vi "Convert Array to ImprocOptions.vi"(1 "Array":i32[](array[numeric])) -> (0 "IMPROCOPTIONS":T1 {"FilterCode" items=["PREWITT_3X3_V"=1, "PREWITT_3X3_H"=2, "SOBEL_3X3_V"=3, "SOBEL_3X3_H"=4, "LAPLACIAN_3X3"=5, "LAPLACIAN_5X5"=6, "GAUSSIAN_3X3"=7, "GAUSSIAN_5X5"=8, "HIPASS_3x3"=9, "HIPASS_5x5"=10, "SHARPEN_3X3"=11, "USERFILTER"=-1]; "Rotate" min=-90 max=90 step=1; "Saturation" min=-100 max=100 step=1; "Contrast" min=-100 max=100 step=1; "Bright" min=-100 max=100 step=1})   [LabVIEW 2013, in "VRI.lvlib"]
uses:
  VRI.lvlib
  _Type Defs/PhInt IMPROCOPTIONS.ctl
  _Type Defs/PhInt WBGAIN.ctl
  _Type Defs/FilterCode.ctl
  _Type Defs/IMFILTER.ctl
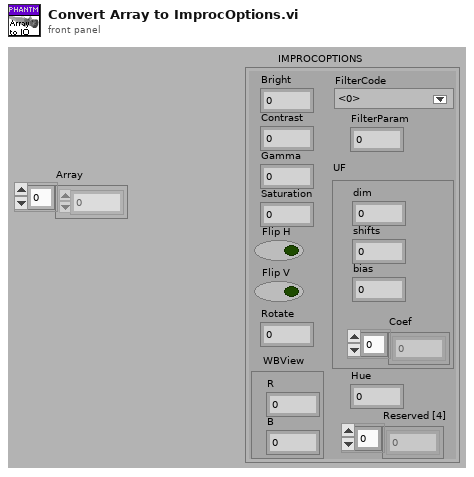
[diagram p1: front panel]
types:
  T1 = typedef "VRI.lvlib/PhInt IMPROCOPTIONS.ctl" = cluster{"Bright":i32, "Contrast":i32, "Gamma":sgl, "Saturation":i32, "Flip H":bool, "Flip V":bool, "Rotate":i32, "WBView":T2, "FilterCode":T3, "FilterParam":i32, "UF":T4, "Hue":i32, "Reserved [4]":i32[]}
  T2 = typedef "VRI.lvlib/PhInt WBGAIN.ctl" = cluster{"R":sgl, "B":sgl}
  T3 = typedef "VRI.lvlib/FilterCode.ctl" = i32
  T4 = typedef "VRI.lvlib/IMFILTER.ctl" = cluster{"dim":i32, "shifts":i32, "bias":i32, "Coef":i32[]}
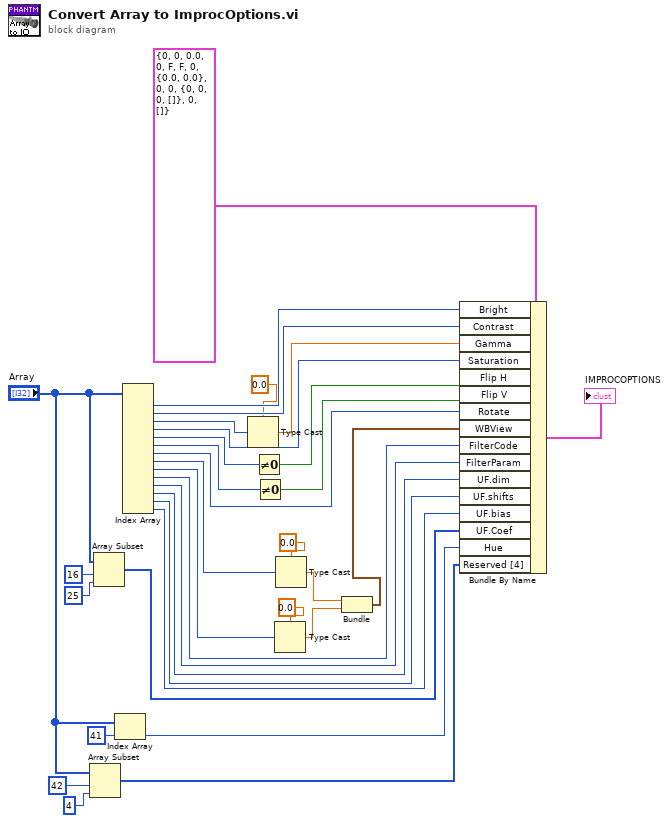
[diagram p0: block diagram]
diagram:
  n1 = Array Subset(array="Array", index=42, length=4) -> (w3:i32[])
  n2 = Array Subset(array="Array", index=16, length=25) -> (w7:i32[])
  n3 = Index Array(array="Array", index=41) -> (element=w6:i32)
  n4 = Index Array(array="Array") -> (element #1=w33:i32, element #2=w32:i32, element #3=w31:i32, element #4=w27:i32, element #5=w26:i32, element #6=w24:i32, element #7=w22:i32, element #8=w20:i32, element #9=w18:i32, element #10=w14:i32, element #11=w13:i32, element #12=w12:i32, element #13=w11:i32, element #14=w10:i32)  [unwired: 14 in]
  n5 = Type Cast(type=sgl 0.0 ("Gamma"), x=w31) -> (*(type *) &x=w30:sgl)
  n6 = Not Equal To 0?(x=w26) -> (x != 0?=w25:bool)
  n7 = Not Equal To 0?(x=w24) -> (x != 0?=w23:bool)
  n8 = Type Cast(type=sgl 0.0 ("Gamma"), x=w18) -> (*(type *) &x=w16:sgl)
  n9 = Type Cast(type=sgl 0.0 ("Gamma"), x=w20) -> (*(type *) &x=w17:sgl)
  n10 = Bundle("Gamma"=w17, "Gamma"=w16) -> (w15:cluster{"Gamma":sgl, "Gamma":sgl})  [unwired: 1 out]
  n11 = Bundle By Name(cluster=T1 {"Bright"=0, "Contrast"=0, "Gamma"=0.0, "Saturation"=0, "Flip H"=FALSE, "Flip V"=FALSE, "Rotate"=0, "WBView"={"R"=0.0, "B"=0.0}, "FilterCode"=0, "FilterParam"=0, "UF"={"dim"=0, "shifts"=0, "bias"=0, "Coef"=[]}, "Hue"=0, "Reserved [4]"=[]} ("IMPROCOPTIONS"), "Bright"=w33, "Contrast"=w32, "Gamma"=w30, "Saturation"=w27, "Flip H"=w25, "Flip V"=w23, "Rotate"=w22, "WBView"=w15, "FilterCode"=w14, "FilterParam"=w13, "UF.dim"=w12, "UF.shifts"=w11, "UF.bias"=w10, "UF.Coef"=w7, "Hue"=w6, "Reserved [4]"=w3) -> (→"IMPROCOPTIONS":T1)
